vi "Encode ACW Parameters.vi"(6 "scanner?":bool, 8 "ADD Parameters (in)":string, 9 "Scanner Settings":T2={"Scan1"=1, "Scan2"=1, "Scan3"=1, "Scan4"=1, "Scan5"=1, "Scan6"=1, "Scan7"=1, "Scan8"=1, "Scan9"=1, "Scan10"=1, "Scan11"=1, "Scan12"=1, "Scan13"=1, "Scan14"=1, "Scan15"=1, "Scan16"=1} {"Scan16" scale=0.0..2.0; "Scan15" scale=0.0..2.0; "Scan14" scale=0.0..2.0; "Scan13" scale=0.0..2.0; "Scan12" scale=0.0..2.0; "Scan11" scale=0.0..2.0; "Scan10" scale=0.0..2.0; "Scan9" scale=0.0..2.0; "Scan8" scale=0.0..2.0; "Scan7" scale=0.0..2.0; "Scan6" scale=0.0..2.0; "Scan5" scale=0.0..2.0; "Scan4" scale=0.0..2.0; "Scan3" min=0 max=2 scale=0.0..2.0; "Scan2" min=0 max=2 scale=0.0..2.0; "Scan1" min=0 max=2 scale=0.0..2.0}, 11 "ACW Test Parameters in":T1={"Voltage (1240)"=1240, "High Limit Total (10)"=5.0, "Low Limit Total (0)"=0.0, "High Limit Real(10)"=10.0, "Low Limit Real (0)"=0.0, "Ramp Up Time (0.1 - 999.9 seconds) (0.1)"=0.1, "Dwell Time (0, 0.2 - 999.9 seconds) (1)"=1.0, "Ramp Down Time (0.0 - 999.9 seconds) (1)"=0.0, "Arc Sense (1 - 9) (5)"=5, "Arc Detect (F: Off)"=FALSE, "Continuity (F: Off)"=FALSE, "Range  "=enum."AUTO", "Offset (0)"=0.0, "Auto Offset (F: Off)"=FALSE, "Frequency"=enum."60"} {"Offset (0)" format="%.2f"; "Ramp Down Time (0.0 - 999.9 seconds) (1)" format="%.1f"; "Low Limit Real (0)" format="%.3f"; "High Limit Real(10)" format="%.2f"; "Dwell Time (0, 0.2 - 999.9 seconds) (1)" format="%.1f"; "Ramp Up Time (0.1 - 999.9 seconds) (0.1)" format="%.1f"; "Low Limit Total (0)" format="%.3f"; "High Limit Total (10)" format="%.2f"; "Voltage (1240)" min=0 max=12000}) -> (0 "Scanner Settings out":T2={"Scan1"=1, "Scan2"=1, "Scan3"=1, "Scan4"=1, "Scan5"=1, "Scan6"=1, "Scan7"=1, "Scan8"=1, "Scan9"=1, "Scan10"=1, "Scan11"=1, "Scan12"=1, "Scan13"=1, "Scan14"=1, "Scan15"=1, "Scan16"=1} {"Scan16" scale=0.0..2.0; "Scan15" scale=0.0..2.0; "Scan14" scale=0.0..2.0; "Scan13" scale=0.0..2.0; "Scan12" scale=0.0..2.0; "Scan11" scale=0.0..2.0; "Scan10" scale=0.0..2.0; "Scan9" scale=0.0..2.0; "Scan8" scale=0.0..2.0; "Scan7" scale=0.0..2.0; "Scan6" scale=0.0..2.0; "Scan5" scale=0.0..2.0; "Scan4" scale=0.0..2.0; "Scan3" min=0 max=2 scale=0.0..2.0; "Scan2" min=0 max=2 scale=0.0..2.0; "Scan1" min=0 max=2 scale=0.0..2.0}, 2 "ACW Test Parameters Out":T1={"Voltage (1240)"=1240, "High Limit Total (10)"=5.0, "Low Limit Total (0)"=0.0, "High Limit Real(10)"=10.0, "Low Limit Real (0)"=0.0, "Ramp Up Time (0.1 - 999.9 seconds) (0.1)"=0.1, "Dwell Time (0, 0.2 - 999.9 seconds) (1)"=1.0, "Ramp Down Time (0.0 - 999.9 seconds) (1)"=0.0, "Arc Sense (1 - 9) (5)"=5, "Arc Detect (F: Off)"=FALSE, "Continuity (F: Off)"=FALSE, "Range  "=enum."AUTO", "Offset (0)"=0.0, "Auto Offset (F: Off)"=FALSE, "Frequency"=enum."60"} {"Offset (0)" format="%.2f"; "Ramp Down Time (0.0 - 999.9 seconds) (1)" format="%.1f"; "Low Limit Real (0)" format="%.3f"; "High Limit Real(10)" format="%.2f"; "Dwell Time (0, 0.2 - 999.9 seconds) (1)" format="%.1f"; "Ramp Up Time (0.1 - 999.9 seconds) (0.1)" format="%.1f"; "Low Limit Total (0)" format="%.3f"; "High Limit Total (10)" format="%.2f"; "Voltage (1240)" min=0 max=12000}, 3 "ADD Parameters":string)   [LabVIEW 2020, in "Associated Research 78XX Series.lvlib"]
uses:
  <instrlib>/Associated Research 78XX Series/Associated Research 78XX Series.lvlib
  <instrlib>/Associated Research 78XX Series/Public/Configure/Steps/Low Level/Scanner Settings.ctl
  <instrlib>/Associated Research 78XX Series/Public/Configure/Steps/Low Level/ACW Test Parameters.ctl
panel:
  # "On\nOff"
  # "On\nOff"
  # "On\nOff"
  # "On\nOff"
  # "On\nOff"
  # "On\nOff"
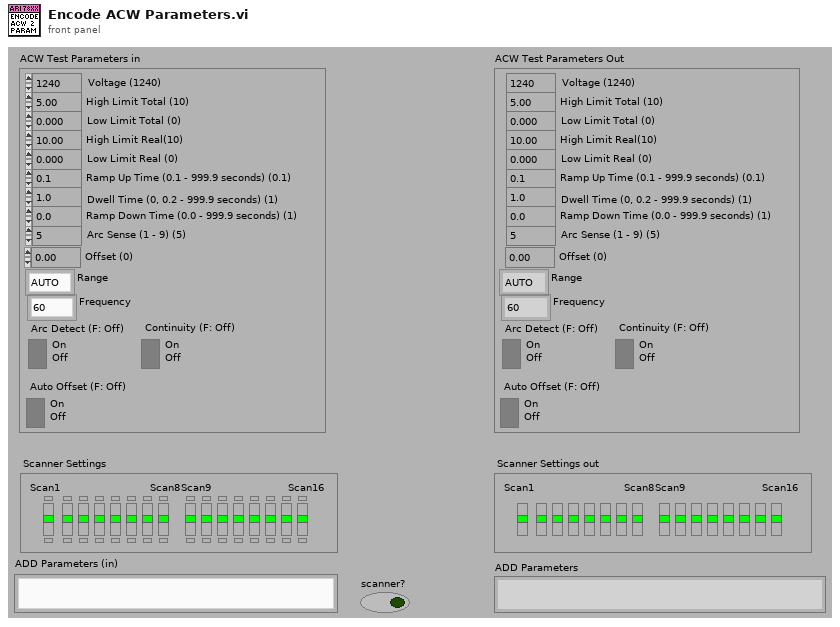
[diagram p1: front panel]
types:
  T1 = typedef "Associated Research 78XX Series.lvlib/ACW Test Parameters.ctl" = cluster{"Voltage (1240)":i32, "High Limit Total (10)":dbl, "Low Limit Total (0)":dbl, "High Limit Real(10)":dbl, "Low Limit Real (0)":dbl, "Ramp Up Time (0.1 - 999.9 seconds) (0.1)":dbl, "Dwell Time (0, 0.2 - 999.9 seconds) (1)":dbl, "Ramp Down Time (0.0 - 999.9 seconds) (1)":dbl, "Arc Sense (1 - 9) (5)":i32, "Arc Detect (F: Off)":bool, "Continuity (F: Off)":bool, "Range  ":enum16{"AUTO", "FIXED"}, "Offset (0)":dbl, "Auto Offset (F: Off)":bool, "Frequency":enum16{"50", "60", "400", "800"}}
  T2 = typedef "Associated Research 78XX Series.lvlib/Scanner Settings.ctl" = cluster{"Scan1":i32, "Scan2":i32, "Scan3":i32, "Scan4":i32, "Scan5":i32, "Scan6":i32, "Scan7":i32, "Scan8":i32, "Scan9":i32, "Scan10":i32, "Scan11":i32, "Scan12":i32, "Scan13":i32, "Scan14":i32, "Scan15":i32, "Scan16":i32}
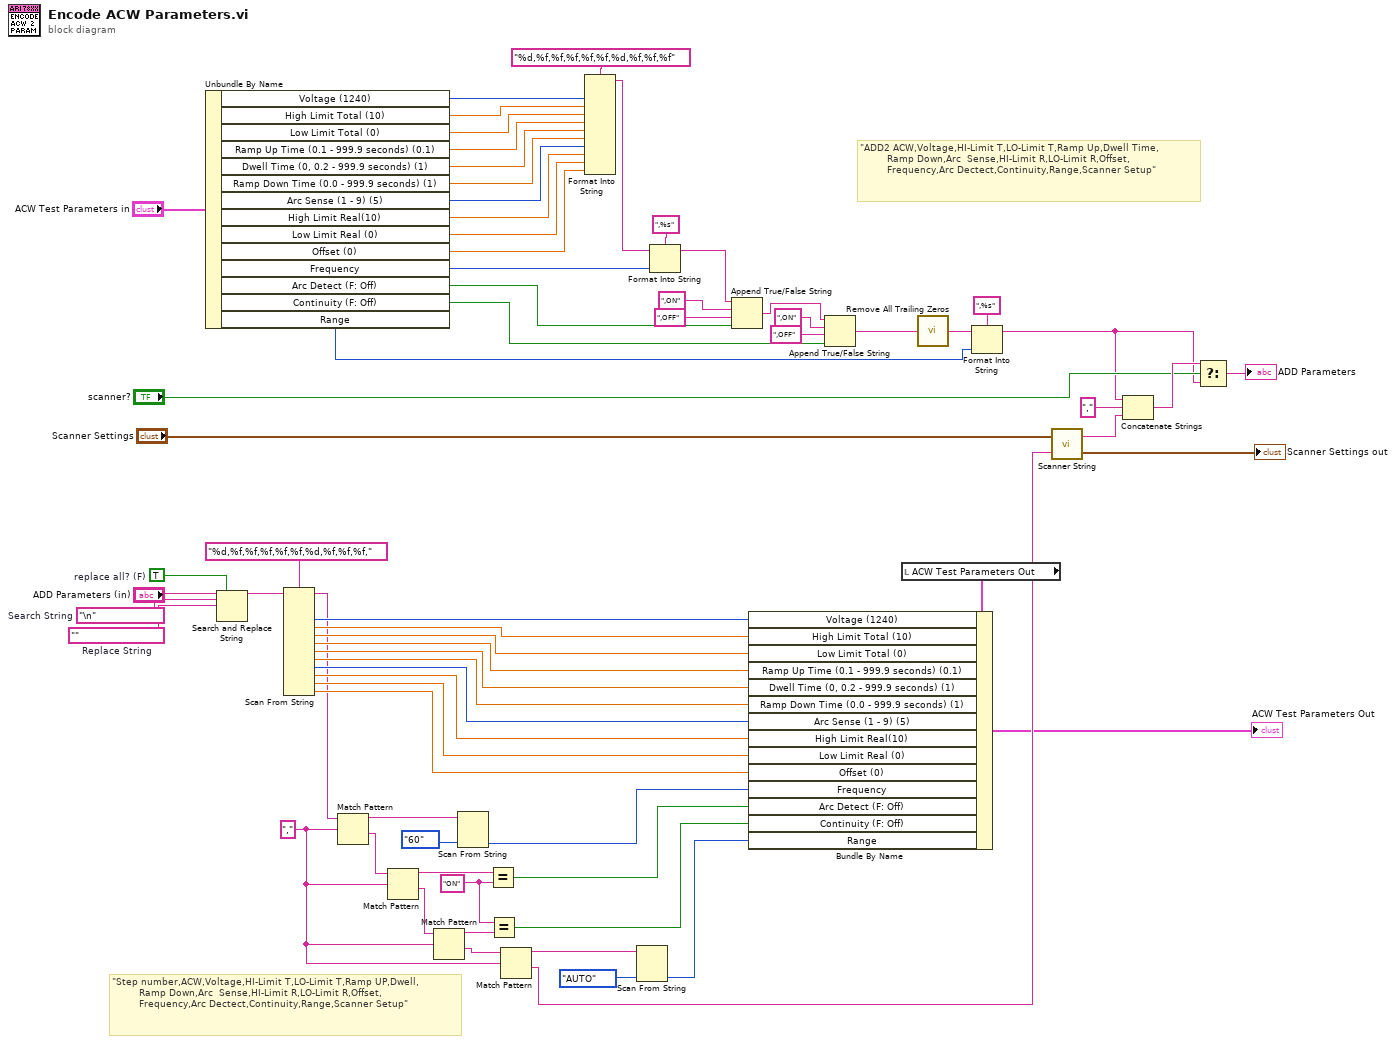
[diagram p0: block diagram]
diagram:
  w40 = TRUE  # replace all? (F)
  w41 = ""  # Replace String
  w42 = "\n"  # Search String
  w44 = "ON" ("y")
  w6 = "," ("regular expression")
  # "\"Step number,ACW,Voltage,HI-Limit T,LO-Limit T,Ramp UP,Dwell,\n         Ramp Down,Arc  Sense,HI-Limit R,LO-Limit R,Offset,\n         Frequency,Arc Dectect,Continuity,Range,Scanner Setup\""
  # "\"ADD2 ACW,Voltage,HI-Limit T,LO-Limit T,Ramp Up,Dwell Time,\n         Ramp Down,Arc  Sense,HI-Limit R,LO-Limit R,Offset,\n         Frequency,Arc Dectect,Continuity,Range,Scanner Setup\""
  n1 = Unbundle By Name("ACW Test Parameters in") -> ("Voltage (1240)"=w43:i32, "High Limit Total (10)"=w21:dbl, "Low Limit Total (0)"=w30:dbl, "Ramp Up Time (0.1 - 999.9 seconds) (0.1)"=w70:dbl, "Dwell Time (0, 0.2 - 999.9 seconds) (1)"=w69:dbl, "Ramp Down Time (0.0 - 999.9 seconds) (1)"=w68:dbl, "Arc Sense (1 - 9) (5)"=w67:i32, "High Limit Real(10)"=w22:dbl, "Low Limit Real (0)"=w66:dbl, "Offset (0)"=w33:dbl, "Frequency"=w9:enum16{"50", "60", "400", "800"}, "Arc Detect (F: Off)"=w65:bool, "Continuity (F: Off)"=w64:bool, "Range"=w29:enum16{"AUTO", "FIXED"})
  n2 = Search and Replace String(replace all?=w40, input string="ADD Parameters (in)", search string=w42, replace string=w41) -> (result string=w38:string)  [unwired: 4 in, 3 out]
  n3 = Scan From String(format string="%d,%f,%f,%f,%f,%f,%d,%f,%f,%f," ("Format String"), input string=w38) -> (remaining string=w5:string, output 1=w60:i32, output 2=w59:dbl, output 3=w58:dbl, output 4=w57:dbl, output 5=w56:dbl, output 6=w55:dbl, output 7=w54:i32, output 8=w53:dbl, output 9=w52:dbl, output 10=w32:dbl)  [unwired: 12 in, 2 out]
  n4 = Match Pattern(string=w5, regular expression=w6) -> (before substring=w3:string, after substring=w4:string)  [unwired: 1 in, 2 out]
  n5 = Match Pattern(string=w4, regular expression=w6) -> (before substring=w51:string, after substring=w48:string)  [unwired: 1 in, 2 out]
  n6 = Match Pattern(string=w48, regular expression=w6) -> (before substring=w47:string, after substring=w34:string)  [unwired: 1 in, 2 out]
  n7 = Scan From String(input string=w3, default 1=enum16{"50", "60", "400", "800"}."60" ("Frequency")) -> (output 1=w1:enum16{"50", "60", "400", "800"})  [unwired: 3 in, 3 out]
  n8 = Equal?(x=w51, y=w44) -> (x = y?=w49:bool)
  n9 = Equal?(x=w44, y=w47) -> (x = y?=w50:bool)
  n10 = Match Pattern(string=w34, regular expression=w6) -> (before substring=w25:string, after substring=w23:string)  [unwired: 1 in, 2 out]
  n11 = Format Into String(format string="%d,%f,%f,%f,%f,%f,%d,%f,%f,%f" ("Format String"), w43, w21, w30, w70, w69, w68, w67, w22, w66, w33) -> (resulting string=w8:string)  [unwired: 2 in, 1 out]
  n12 = Scan From String(input string=w25, default 1=enum16{"AUTO", "FIXED"}."AUTO" ("Enum")) -> (output 1=w24:enum16{"AUTO", "FIXED"})  [unwired: 3 in, 3 out]
  n13 = Format Into String(format string=",%s", initial string=w8, w9) -> (resulting string=w7:string)  [unwired: 1 in, 1 out]
  n14 = Append True/False String(1:w65, 2:",OFF" ("false string"), 3:",ON" ("true string"), 4:w7) -> (0:w11:string)
  n15 = Append True/False String(1:w64, 2:",OFF" ("false string"), 3:",ON" ("true string"), 4:w11) -> (0:w37:string)
  n16 = local read "ACW Test Parameters Out"() -> (w14:T1)
  n17 = Bundle By Name(cluster=w14, "Voltage (1240)"=w60, "High Limit Total (10)"=w59, "Low Limit Total (0)"=w58, "Ramp Up Time (0.1 - 999.9 seconds) (0.1)"=w57, "Dwell Time (0, 0.2 - 999.9 seconds) (1)"=w56, "Ramp Down Time (0.0 - 999.9 seconds) (1)"=w55, "Arc Sense (1 - 9) (5)"=w54, "High Limit Real(10)"=w53, "Low Limit Real (0)"=w52, "Offset (0)"=w32, "Frequency"=w1, "Arc Detect (F: Off)"=w49, "Continuity (F: Off)"=w50, "Range"=w24) -> (→"ACW Test Parameters Out":T1)
  n18 = call <instrlib>:"Remove All Trailing Zeros.vi"("String in"=w37) -> ("String out"=w26:string)
  n19 = Format Into String(format string=",%s", initial string=w26, w29) -> (resulting string=w27:string)  [unwired: 1 in, 1 out]
  n20 = call <instrlib>:"Scanner String.vi"("Scanner String (in)"=w23, "Scanner Settings in"="Scanner Settings") -> ("Scanner Settings out"=→"Scanner Settings out":T2, "Scanner String (out)"=w36:string)
  n21 = Concatenate Strings(w27, "," ("Substring"), w36) -> (w35:string)
  n22 = Select(t=w35, s="scanner?", f=w27) -> (s? t:f=→"ADD Parameters":string)
